vi "PR Serial Number.vi"() -> (0 "Serial Number":string)   [LabVIEW 2023, in "BS6006PRPLUS.lvlib"]
doc: "The function gets the serial number of the pulser/receiver which is connected.\n\n\n\nextern \"C\" BS6006PRPLUS_API void __cdecl PR_SerialNumber(char *SN);\nextern \"C\" BS6006PRPLUS_API char* __cdecl PR_SerialNumber();"
uses:
  BS6006PRPLUS.lvlib
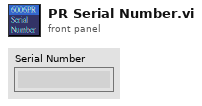
[diagram p1: front panel]
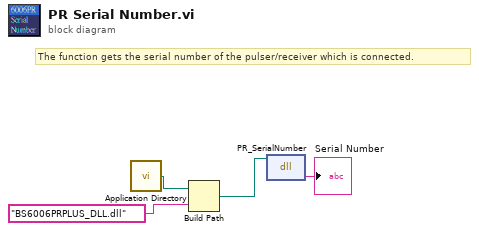
[diagram p0: block diagram]
diagram:
  # "The function gets the serial number of the pulser/receiver which is connected."
  n1 = call <vilib>:"Application Directory.vi"() -> ("Application Directory"=w3:path)
  n2 = Build Path(base path=w3, name or relative path="BS6006PRPLUS_DLL.dll") -> (appended path=w1:path)
  n3 = dll-call lib="E:/Broadsound_Program/PulserReceiver/6006PR PLUS/API/DLL/LabVIEW 15/VIs/BS6006PRPLUS_DLL.dlls" fn="PR_SerialNumber"(path in=w1) -> ("return type"=→"Serial Number":string)  [unwired: 2 in, 2 out]
